vi "read_img_data.vi"(7 "error in (no error)":errorcluster, 10 "Input path":path) -> (0 "error out":errorcluster, 2 "Image Out":T1, 3 "Output path":path)   [LabVIEW 2020]
uses:
  <vilib>/vision/Image Controls.llb/IMAQ Image.ctl
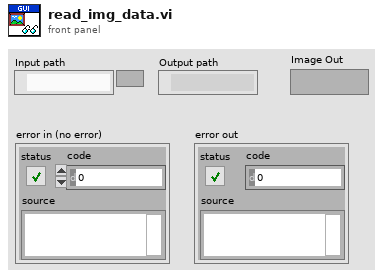
[diagram p1: front panel]
types:
  T1 = typedef "IMAQ Image.ctl" = refnum<image>
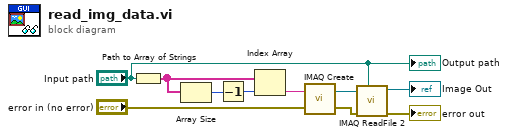
[diagram p0: block diagram]
diagram:
  n1 = Path to Array of Strings(0:"Input path") -> (2:w10:string[])  [unwired: 1 out]
  n2 = Array Size(array=w10) -> (size(s)=w9:i32)
  n3 = Decrement(x=w9) -> (x-1=w8:i32)
  n4 = Index Array(array=w10, index=w8) -> (element=w7:string)
  n5 = call "IMAQ Create"("Image Name"=w7, "error in (no error)"="error in (no error)") -> ("New Image"=w5:T1, "error out"=w4:errorcluster)  [unwired: 3 in]
  n6 = call "IMAQ ReadFile 2"("File Path"="Input path", "error in (no error)"=w4, "Image"=w5) -> ("error out"=→"error out":errorcluster, "Image Out"=→"Image Out":T1)  [unwired: 4 in, 3 out]
  "Output path" <- "Input path"
